vi "Test.vi"   [LabVIEW 2016]
doc: "This VI is called when test mode begins, and will automatically be terminated when it ends. You can add manual or automatic tests and invoke them from the dashboard."
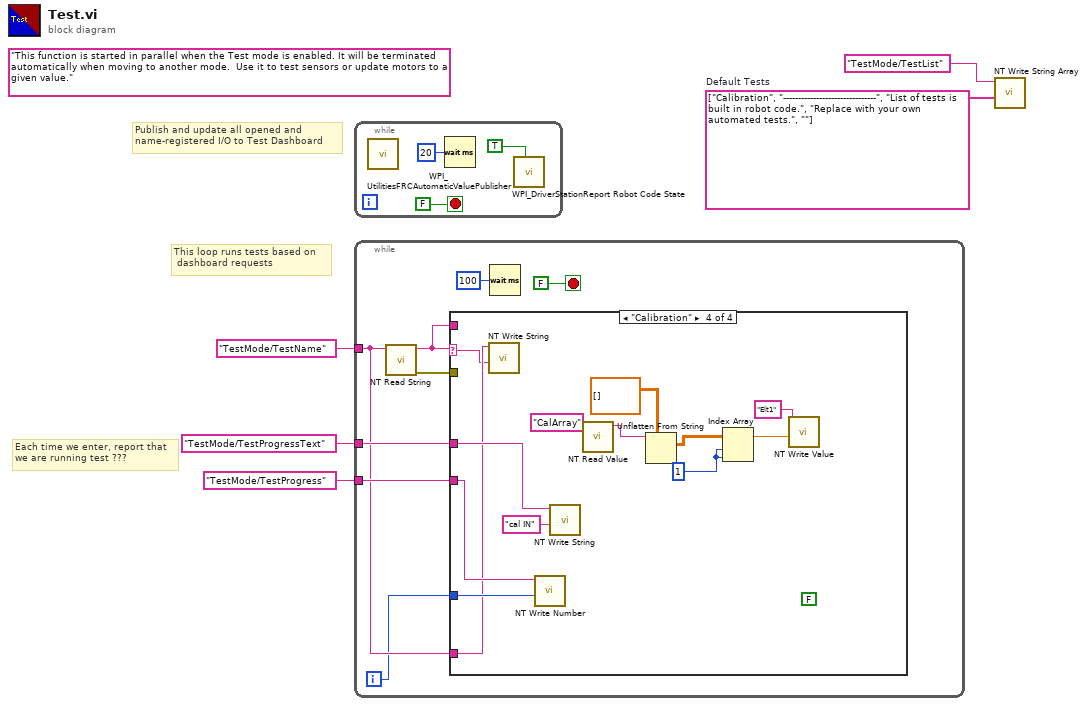
[diagram p0: block diagram]
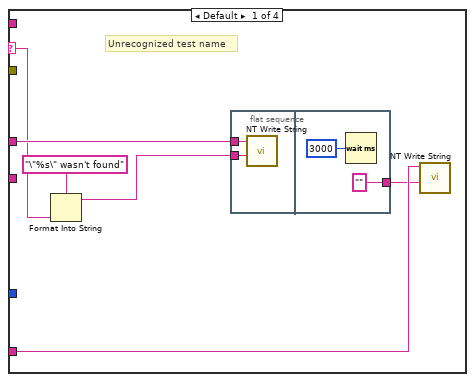
[diagram p2: hidden frame]
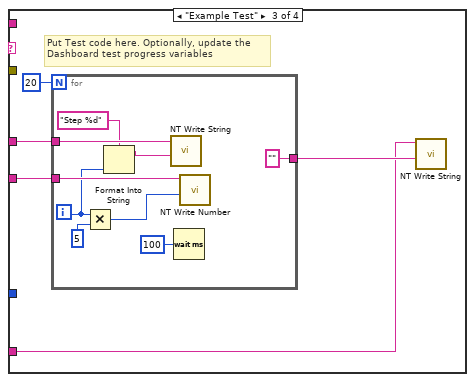
[diagram p4: hidden frame]
diagram:
  w2 = string[] ["Calibration", "-------------------------------", "List of tests is built in robot code.", "Replace with your own automated tests.", ""]  # Default Tests
  (unwired) "This function is started in parallel when the Test mode is enabled. It will be terminated automatically when moving to another mode.  Use it to test sensors or update motors to a given value."
  # "This loop runs tests based on \n dashboard requests"
  # "Publish and update all opened and\nname-registered I/O to Test Dashboard"
  # "Each time we enter, report that\nwe are running test ???"
  n1 = while {
    stop <- FALSE stop-if-true
    n2 = call <vilib>:"WPI_UtilitiesFRCAutomaticValuePublisher.vi"() -> ()  [unwired: 12 in]
    n3 = Wait (ms)(milliseconds to wait=u32 20) -> ()  [unwired: 1 out]
    n4 = call <vilib>:"WPI_DriverStationReport Robot Code State.vi"("Test"=TRUE ("Autonomous")) -> ()  [unwired: 10 in, 1 out]
  }
  n5 = while {
    tunnel: "TestMode/TestName" ("Name") -> [w11]
    tunnel: "TestMode/TestProgressText" ("Name") -> [w14]
    tunnel: "TestMode/TestProgress" ("Name") -> [w13]
    i -> [w9]
    stop <- FALSE stop-if-true
    n6 = call <vilib>:"NT Read String.vi"("Name"=w11) -> ("error out"=w10:errorcluster, "String"=w12:string)  [unwired: 9 in]
    n7 = case shown="\"Calibration\"" w12 {
      selector: w12 -> [w21 _ _ w41]
      tunnel: w11 -> [w18 _ w27 w42]
      tunnel: w14 -> [w22 _ w30 w46]
      tunnel: w13 -> [_ _ w31 w44]
      tunnel: w12 -> [_ _ _ _]
      tunnel: w10 -> [_ _ _ _]
      tunnel: w9 -> [_ _ _ w43]
      frame Default {
        # "Unrecognized test name"
        n8 = Format Into String(format string="\"%s\" wasn't found" ("Name"), w21) -> (resulting string=w20:string)  [unwired: 2 in, 1 out]
        n9 = flat-sequence {
          tunnel: w22 -> [w23]
          tunnel: w20 -> [w24]
          tunnel: ["" ("Name")] -> w17
          frame #0 {
            n10 = call <vilib>:"NT Write String.vi"("String"=w24, "Name"=w23) -> ()  [unwired: 9 in, 1 out]
          }
          frame #1 {
            n11 = Wait (ms)(milliseconds to wait=u32 3000) -> ()  [unwired: 1 out]
          }
        }
        n12 = call <vilib>:"NT Write String.vi"("String"=w17, "Name"=w18) -> ()  [unwired: 9 in, 1 out]
      }
      frame "" {
        # "No test to run"
      }
      frame "Example Test" {
        # "Put Test code here. Optionally, update the\nDashboard test progress variables"
        n13 = for {
          N: 20 -> [_]
          tunnel: w31 -> [w40]
          tunnel: w30 -> [w38]
          tunnel: ["" ("String")] -> w28
          i -> [w35]
          n14 = Multiply(x=w35, y=u32 5 ("milliseconds to wait")) -> (x*y=w36:u32)
          n15 = Format Into String(format string="Step %d", w35) -> (resulting string=w33:string)  [unwired: 2 in, 1 out]
          n16 = call <vilib>:"NT Write String.vi"("String"=w33, "Name"=w38) -> ()  [unwired: 9 in, 1 out]
          n17 = Wait (ms)(milliseconds to wait=u32 100) -> ()  [unwired: 1 out]
          n18 = call <vilib>:"NT Write Number.vi"("Numeric"=w36, "Name"=w40) -> ()  [unwired: 9 in, 1 out]
        }
        n19 = call <vilib>:"NT Write String.vi"("String"=w28, "Name"=w27) -> ()  [unwired: 9 in, 1 out]
      }
      frame "Calibration" {
        w47 = 1 ("index")
        (unwired) FALSE
        n20 = call <vilib>:"NT Write String.vi"("String"=w41, "Name"=w42) -> ()  [unwired: 9 in, 1 out]
        n21 = call <vilib>:"NT Write Number.vi"("Numeric"=w43, "Name"=w44) -> ()  [unwired: 9 in, 1 out]
        n22 = call <vilib>:"NT Write String.vi"("String"="cal IN", "Name"=w46) -> ()  [unwired: 9 in, 1 out]
        n23 = call-poly <vilib>:"NT Read Value.vi"("Name"="CalArray") -> ("String"=w52:string)  [unwired: 9 in, 1 out]
        n24 = Unflatten From String(type=dbl[][] [], binary string=w52) -> (value=w48:dbl[][])  [unwired: 3 in, 2 out]
        n25 = Index Array(array=w48, index (row)=w47, index (col)=w47) -> (element=w51:dbl)
        n26 = call-poly <vilib>:"NT Write Value.vi"("Numeric"=w51, "Name"="Elt1") -> ()  [unwired: 9 in, 1 out]
      }
    }
    n27 = Wait (ms)(milliseconds to wait=u32 100) -> ()  [unwired: 1 out]
  }
  n28 = call <vilib>:"NT Write String Array.vi"("String Array"=w2, "Name"="TestMode/TestList") -> ()  [unwired: 9 in, 1 out]
